vi "Non Uniform Correction.vi"(8 "error in (no error)":errorcluster, 11 "Flir A700 in":refnum<class "Flir A700.lvclass">) -> (0 "error out":errorcluster, 3 "Flir A700 out":refnum<class "Flir A700.lvclass">)   [LabVIEW 2023, in "HAL.lvlib" / "FLIR A700.lvlib" / "Flir A700.lvclass"]
uses:
  Flir A700.lvclass
  Flir A700.lvclass/Flir A700.ctl
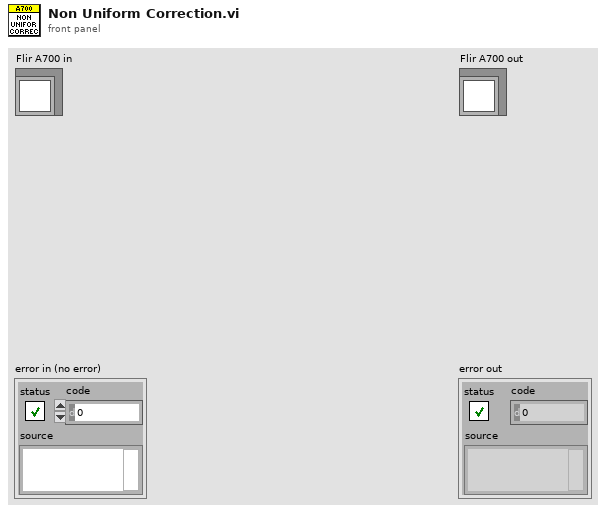
[diagram p1: front panel]
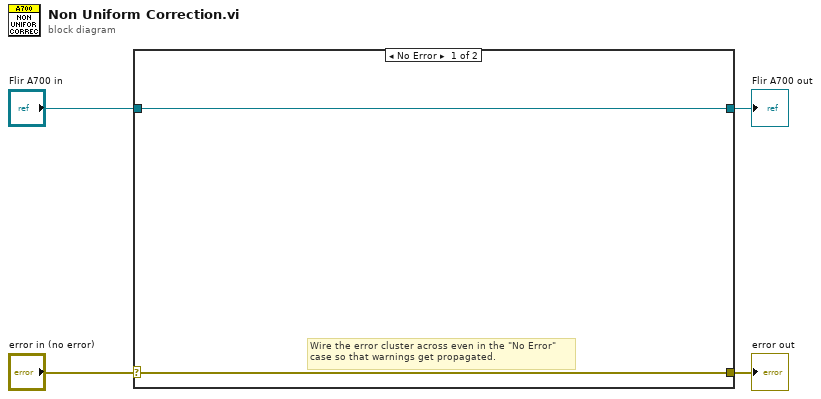
[diagram p0: block diagram]
diagram:
  n1 = case shown="No Error" "error in (no error)" {
    selector: "error in (no error)" -> [w5 w8]
    tunnel: [w5 w8] -> w3
    tunnel: [w6 w7] -> w1
    tunnel: "Flir A700 in" -> [w6 w7]
    frame No Error {
      # "Wire the error cluster across even in the \"No Error\"\ncase so that warnings get propagated."
    }
    frame Error {
    }
  }
  "error out" <- w3
  "Flir A700 out" <- w1
